vi "isPlaying.vi"() -> ()   [LabVIEW 2014]
panel:
  out "AllBellsShouldStop":bool
  out "15mBellShouldStop":bool
  out "35mBellShouldStop":bool
  out "50mBellShouldStop":bool
  out "Count":dbl
  out "isSoundPlaying":bool
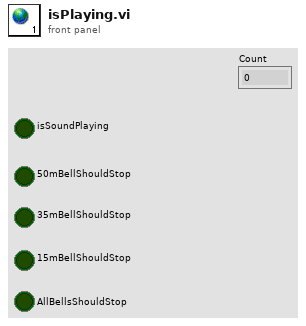
[diagram p1: front panel]
diagram:
